vi "Teleop.vi"(10 "Match Info":T1={"Autonomous Elapsed Seconds"=0.0, "TeleOp Elapsed Seconds"=0.0, "Disabled Elapsed Seconds"=0.0, "Visited Autonomous"=FALSE, "Visited TeleOp"=FALSE, "Visited Disabled"=FALSE, "Autonomous Settings"={"Autonomous Style"=enum."Independent", "VI Refnum"=refnum}}, 11 "Call Context":T2) -> ()   [LabVIEW 2015]
doc: "This VI is called for each TeleOp packet received from the DS where the robot is not disabled. It is often used to read from the joysticks and update I/O or to update setpoints for timed control loops. It should complete and return within 20 milliseconds or it may miss DS packets."
uses:
  <vilib>/Rock Robotics/WPI/DriverStation/WPI_DriverStationDerivedRobotMode.ctl
  <vilib>/Rock Robotics/WPI/DriverStation/WPI_DriverStationMatch Info.ctl
  <vilib>/Rock Robotics/Network Tables/SD Read Boolean.vi
  <vilib>/Rock Robotics/Network Tables/SD Read Number.vi
  <vilib>/Rock Robotics/WPI/Utilities/WPI_GetSetVariantRefNum.vi
panel:
  out "final_test":dbl
  out "test":dbl
  out "Sample Slider 0":dbl(slide) scale=0.0..5.0
  out "Sample Boolean 1":bool
  out "Sample Boolean 0":bool
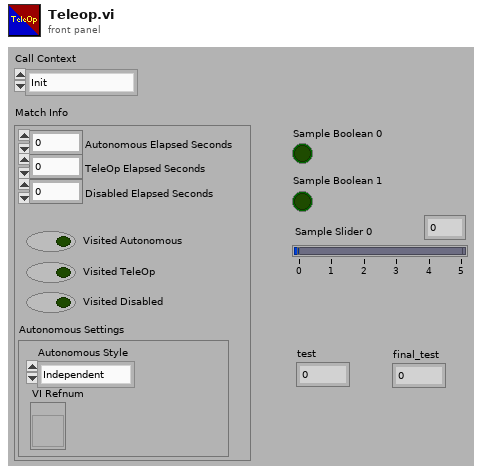
[diagram p1: front panel]
types:
  T1 = typedef "WPI_DriverStationMatch Info.ctl" = cluster{"Autonomous Elapsed Seconds":dbl, "TeleOp Elapsed Seconds":dbl, "Disabled Elapsed Seconds":dbl, "Visited Autonomous":bool, "Visited TeleOp":bool, "Visited Disabled":bool, "Autonomous Settings":cluster{"Autonomous Style":enum16{"Iterative", "Independent"}, "VI Refnum":refnum<vi>}}
  T2 = typedef "WPI_DriverStationDerivedRobotMode.ctl" = enum16{"Init", "Execute", "Stop"}
  T3 = typedef "WPI_JoystickDevRef.ctl" = cluster{"Device":T4}
  T4 = typedef "WPI_JoystickDeviceEnum.ctl" = enum16{"USB 0", "USB 1", "USB 2", "USB 3", "USB 4", "USB 5"}
  T5 = typedef "WPI_RobotDriveDevRef.ctl" = cluster{"DevStatus":errorcluster, "Motors[]":T6[], "Square Inputs":bool, "Max Output":dbl}
  T6 = typedef "WPI_MotorControlDeviceRef.ctl" = cluster{"DeviceStatus":errorcluster, "Type":T7, "PWM":cluster{"PWM Channel":T8, "DeadBand":T9}, "CAN":cluster{"Device Number":u8, "Control Mode":T10, "Semaphore":T11, "Max Vout":dbl, "TalonSRX Control Mode":T12}, "Invert":bool}
  T7 = typedef "WPI_MotorControlType.ctl" = enum16{"PWM", "CAN", "CANTalonSRX"}
  T8 = typedef "FPGA_DIOPWMChannel.ctl" = enum8{"PWM 0", "PWM 1", "PWM 2", "PWM 3", "PWM 4", "PWM 5", "PWM 6", "PWM 7", "PWM 8", "PWM 9", "PWM MXP 0", "PWM MXP 1", "PWM MXP 2", "PWM MXP 3", "PWM MXP 4", "PWM MXP 5", "PWM MXP 6", "PWM MXP 7", "PWM MXP 8", "PWM MXP 9", "Invalid"}
  T9 = typedef "WPI_PWMDeadband.ctl" = cluster{"Name":string, "maxPositivePwm":i32, "minPositivePwm":i32, "centerPwm":i32, "maxNegativePwm":i32, "minNegativePwm":i32, "angularRange":u16}
  T10 = typedef "WPI_CANJaguar_ControlMode.ctl" = enum8{"Percent VBus", "Current", "Speed", "Position", "Voltage"}
  T11 = typedef "Semaphore RefNum" = refnum<k1>
  T12 = typedef "WPI_CANTalonSRX_APIControlMode.ctl" = enum8{"Percent VBus", "Speed", "Position", "Slave", "Unchanged / Invalid", "Voltage Compensation", "Current", "Motion Profile"}
  T13 = cluster{"Buttons[0]":bool, "Buttons[1]":bool, "Buttons[2]":bool, "Buttons[3]":bool, "Buttons[4]":bool, "Buttons[5]":bool, "Buttons[6]":bool, "Buttons[7]":bool, "Buttons[8]":bool}
  T14 = cluster{"Axes[0]":dbl, "Axes[1]":dbl, "Axes[2]":dbl, "Axes[3]":dbl, "Axes[4]":dbl, "Axes[5]":dbl, "Axes[6]":dbl, "Axes[7]":dbl, "Axes[8]":dbl}
  T15 = typedef "WPI_EncoderDevRef.ctl" = cluster{"DevStatus":errorcluster, "EncoderIndex":T16, "CounterIndex":T17, "DistancePerCount":dbl, "Decoding Type":T18}
  T16 = typedef "FPGA_EncoderIdx.ctl" = enum8{"Enc 0", "Enc 1", "Enc 2", "Enc 3", "Enc 4", "Enc 5", "Enc 6", "Enc 7", "Invalid"}
  T17 = typedef "FPGA_CounterCtrSystemIndex.ctl" = enum8{"Ctr 0", "Ctr 1", "Ctr 2", "Ctr 3", "Ctr 4", "Ctr 5", "Ctr 6", "Ctr 7", "Invalid"}
  T18 = typedef "WPI_EncoderType.ctl" = enum16{"1x", "2x", "4x"}
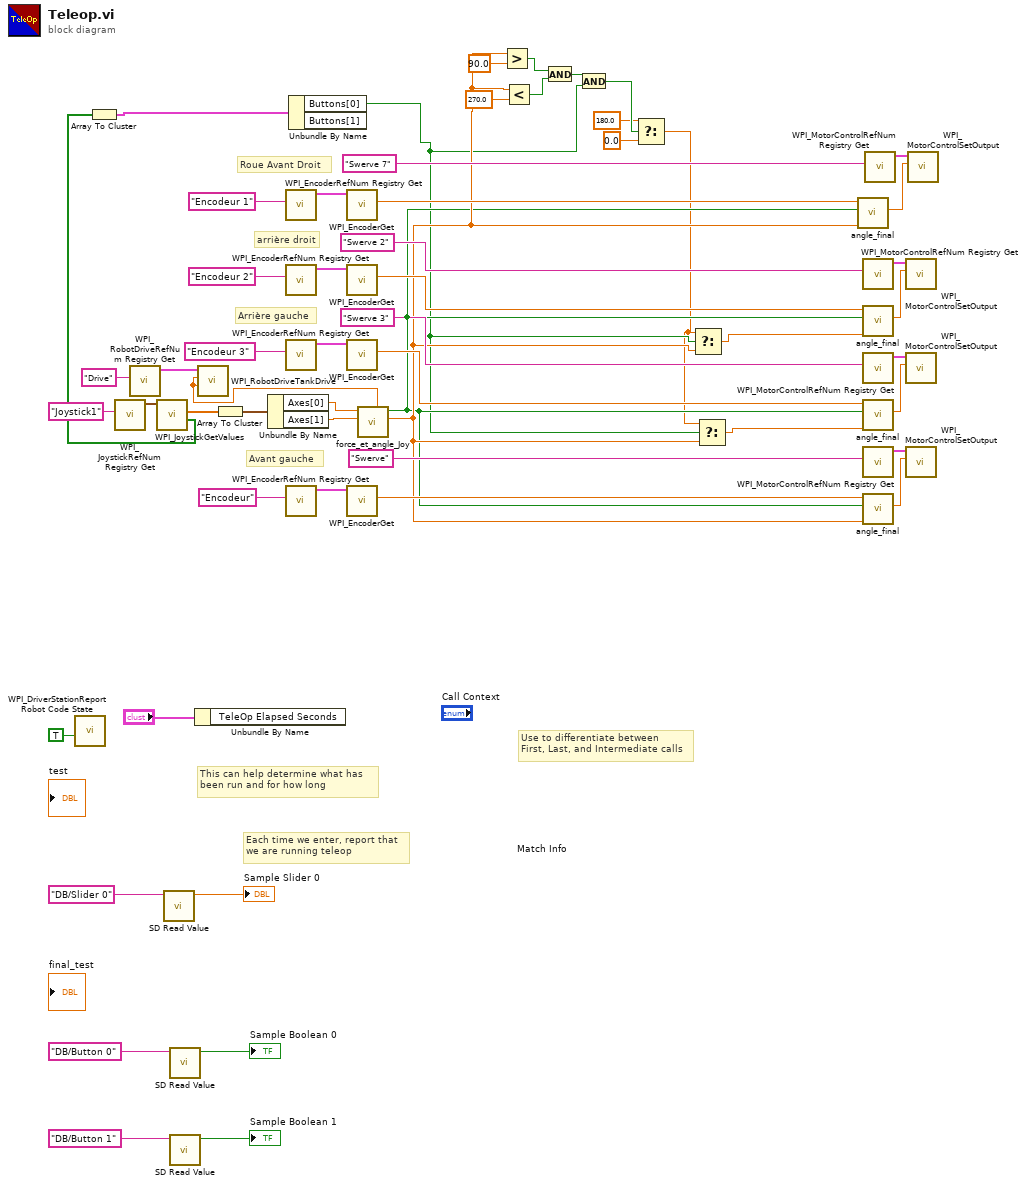
[diagram p0: block diagram]
diagram:
  # "Avant gauche"
  # "Arrière gauche"
  # "arrière droit"
  # "Roue Avant Droit"
  # "Each time we enter, report that\nwe are running teleop"
  # "Use to differentiate between\nFirst, Last, and Intermediate calls"
  # "This can help determine what has\nbeen run and for how long"
  n1 = call <vilib>:"WPI_DriverStationReport Robot Code State.vi"("TeleOp"=TRUE ("Autonomous")) -> ()  [unwired: 10 in, 1 out]
  n2 = call <vilib>:"WPI_JoystickRefNum Registry Get.vi"("refnum name"="Joystick1") -> ("JoystickDevRef"=w49:T3)  [unwired: 9 in, 1 out]
  n3 = call <vilib>:"WPI_RobotDriveRefNum Registry Get.vi"("refnum name"="Drive") -> ("RobotDriveDevRef"=w40:T5)  [unwired: 9 in, 1 out]
  n4 = call <vilib>:"WPI_JoystickGetValues.vi"("JoystickDevRef"=w49) -> ("Buttons"=w15:bool[], "Axes"=w47:dbl[])  [unwired: 6 in, 3 out]
  n5 = Array To Cluster(array=w15) -> (cluster=w14:T13)
  n6 = call-poly <vilib>:"SD Read Value.vi"("Name"="DB/Slider 0" ("refnum name")) -> ("Numeric"=→"Sample Slider 0":dbl)  [unwired: 8 in, 2 out]
  n7 = call-poly <vilib>:"SD Read Value.vi"("Name"="DB/Button 0" ("refnum name")) -> ("Boolean"=→"Sample Boolean 0":bool)  [unwired: 8 in, 2 out]
  n8 = call-poly <vilib>:"SD Read Value.vi"("Name"="DB/Button 1" ("refnum name")) -> ("Boolean"=→"Sample Boolean 1":bool)  [unwired: 8 in, 2 out]
  n9 = Unbundle By Name("Match Info") -> ()  [unwired: 1 out]
  n10 = Array To Cluster(array=w47) -> (cluster=w46:T14)
  n11 = Unbundle By Name(w46) -> ("Axes[0]"=w29:dbl, "Axes[1]"=w28:dbl)
  n12 = call <vilib>:"WPI_EncoderRefNum Registry Get.vi"("refnum name"="Encodeur 1") -> ("EncoderDevRef"=w38:T15)  [unwired: 9 in, 1 out]
  n13 = call <vilib>:"WPI_EncoderRefNum Registry Get.vi"("refnum name"="Encodeur 2") -> ("EncoderDevRef"=w34:T15)  [unwired: 9 in, 1 out]
  n14 = call <vilib>:"WPI_EncoderRefNum Registry Get.vi"("refnum name"="Encodeur 3") -> ("EncoderDevRef"=w32:T15)  [unwired: 9 in, 1 out]
  n15 = call <vilib>:"WPI_EncoderRefNum Registry Get.vi"("refnum name"="Encodeur") -> ("EncoderDevRef"=w42:T15)  [unwired: 9 in, 1 out]
  n16 = Unbundle By Name(w14) -> ("Buttons[0]"=w6:bool)  [unwired: 1 out]
  n17 = call <vilib>:"WPI_EncoderGet.vi"("EncoderDevRef"=w38) -> ("Distance"=w25:dbl)  [unwired: 5 in, 5 out]
  n18 = call <vilib>:"WPI_EncoderGet.vi"("EncoderDevRef"=w34) -> ("Distance"=w23:dbl)  [unwired: 5 in, 5 out]
  n19 = call <vilib>:"WPI_EncoderGet.vi"("EncoderDevRef"=w32) -> ("Distance"=w21:dbl)  [unwired: 5 in, 5 out]
  n20 = call <vilib>:"WPI_EncoderGet.vi"("EncoderDevRef"=w42) -> ("Distance"=w18:dbl)  [unwired: 5 in, 5 out]
  n21 = call "force_et_angle_Joy.vi"("axe 1"=w28, "axe 2"=w29) -> ("angle"=w12:dbl, "in_dead_zone"=w7:bool, "force"=w5:dbl)  [unwired: 7 in]
  n22 = call <vilib>:"WPI_RobotDriveTankDrive.vi"("Right axis value"=w5, "Left axis value"=w5, "RobotDriveDevRef"=w40) -> ()  [unwired: 6 in, 3 out]
  n23 = Greater?(x=w12, y=90.0) -> (0:w10:bool)
  n24 = Less?(x=w12, y=270.0) -> (x < y?=w9:bool)
  n25 = And(x=w10, y=w9) -> (x .and. y?=w8:bool)
  n26 = And(x=w8, y=w6) -> (x .and. y?=w4:bool)
  n27 = Select(t=180.0, s=w4, f=0.0) -> (s? t:f=w1:dbl)
  n28 = Select(t=w1, s=w6, f=w12) -> (s? t:f=w16:dbl)
  n29 = Select(t=w1, s=w6, f=w12) -> (s? t:f=w17:dbl)
  n30 = call "angle_final.vi"("Valeur joy"=w12, "indeadzone"=w7, "valeur enc"=w25) -> ("valeur"=w24:dbl)  [unwired: 8 in]
  n31 = call <vilib>:"WPI_MotorControlRefNum Registry Get.vi"("refnum name"="Swerve 2") -> ("MotorControlDevRef"=w26:T6)  [unwired: 9 in, 1 out]
  n32 = call "angle_final.vi"("Valeur joy"=w16, "indeadzone"=w7, "valeur enc"=w23) -> ("valeur"=w22:dbl)  [unwired: 8 in]
  n33 = call <vilib>:"WPI_MotorControlRefNum Registry Get.vi"("refnum name"="Swerve 3") -> ("MotorControlDevRef"=w31:T6)  [unwired: 9 in, 1 out]
  n34 = call "angle_final.vi"("Valeur joy"=w17, "indeadzone"=w7, "valeur enc"=w21) -> ("valeur"=w20:dbl)  [unwired: 8 in]
  n35 = call <vilib>:"WPI_MotorControlRefNum Registry Get.vi"("refnum name"="Swerve") -> ("MotorControlDevRef"=w44:T6)  [unwired: 9 in, 1 out]
  n36 = call "angle_final.vi"("Valeur joy"=w12, "indeadzone"=w7, "valeur enc"=w18) -> ("valeur"=w19:dbl)  [unwired: 8 in]
  n37 = call <vilib>:"WPI_MotorControlRefNum Registry Get.vi"("refnum name"="Swerve 7") -> ("MotorControlDevRef"=w36:T6)  [unwired: 9 in, 1 out]
  n38 = call <vilib>:"WPI_MotorControlSetOutput.vi"("Output"=w22, "MotorControlDevRef"=w26) -> ()  [unwired: 7 in, 3 out]
  n39 = call <vilib>:"WPI_MotorControlSetOutput.vi"("Output"=w20, "MotorControlDevRef"=w31) -> ()  [unwired: 7 in, 3 out]
  n40 = call <vilib>:"WPI_MotorControlSetOutput.vi"("Output"=w19, "MotorControlDevRef"=w44) -> ()  [unwired: 7 in, 3 out]
  n41 = call <vilib>:"WPI_MotorControlSetOutput.vi"("Output"=w24, "MotorControlDevRef"=w36) -> ()  [unwired: 7 in, 3 out]
